vi "lab_21-3.vi"() -> ()   [LabVIEW 2014]
uses:
  <vilib>/addons/Multicore Analysis and Sparse Matrix/Statistics/_statistics/Mean (DBL).vi
  <vilib>/Analysis/NI_AALBase.lvlib
  <vilib>/measure/NI_MABase.lvlib
  <instrlib>/Rohde&Schwarz HMC 804x Power Supplies/Rohde&Schwarz HMC 804x Power Supplies.lvlib
  <vilib>/addons/Multicore Analysis and Sparse Matrix/Statistics/NI_MASM_Statistics.lvlib
panel:
  out "TERMOCOP":cluster{dbl[], dbl[]}(graph)
  out "PT100":cluster{dbl[], dbl[]}(graph)
  in  "tempo tot acquisiz":dbl=100.0
  in  "durata ciclo\n acquisizione dt":dbl=0.1
  in  "freq acquiisizione":dbl=1000.0
  out "0- PULSE":cluster{dbl[], dbl[]}(graph)
  in  "freq quadra":dbl=10.0 format="%0.2p"
  in  "amp quadra":dbl=1.0 format="%0.2p"
  out "Waveform Graph 2":waveform(dbl)(graph)={"t0"=timestamp(0 s since 1904-01-01), "dt"=0.001, "Y"=array[1000 elements]}
  in  "amplitude":dbl=10.0 format="%0.2f"
  in  "Durata impulso":dbl=0.5
  in  "Ritardo":dbl=10.0
  in  "durata tot \nsegnale impulso":dbl=20.0
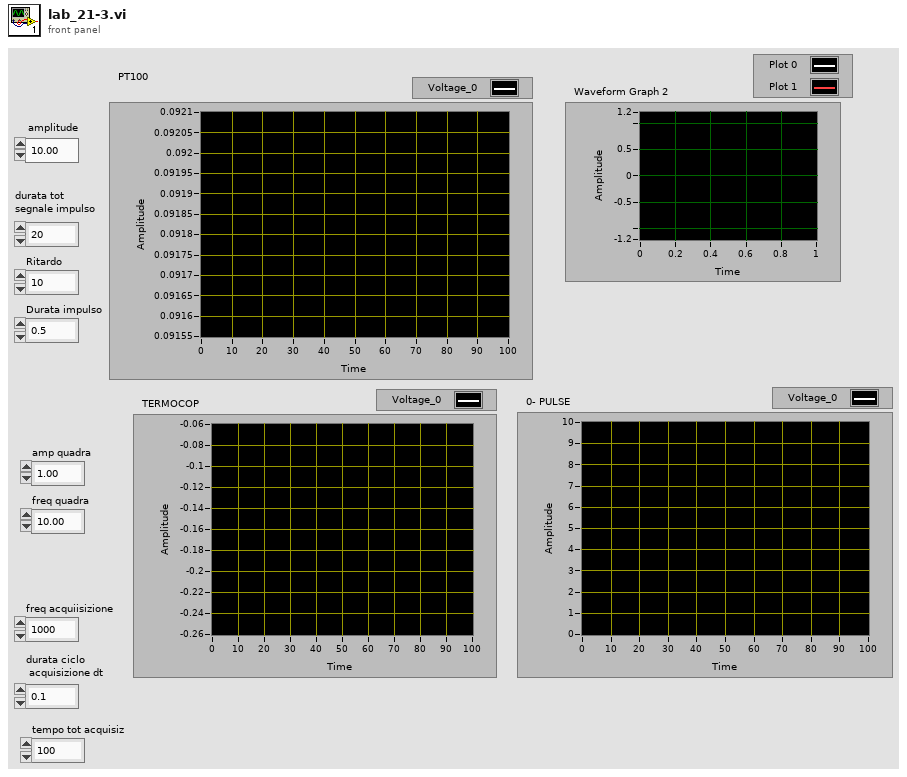
[diagram p1: front panel]
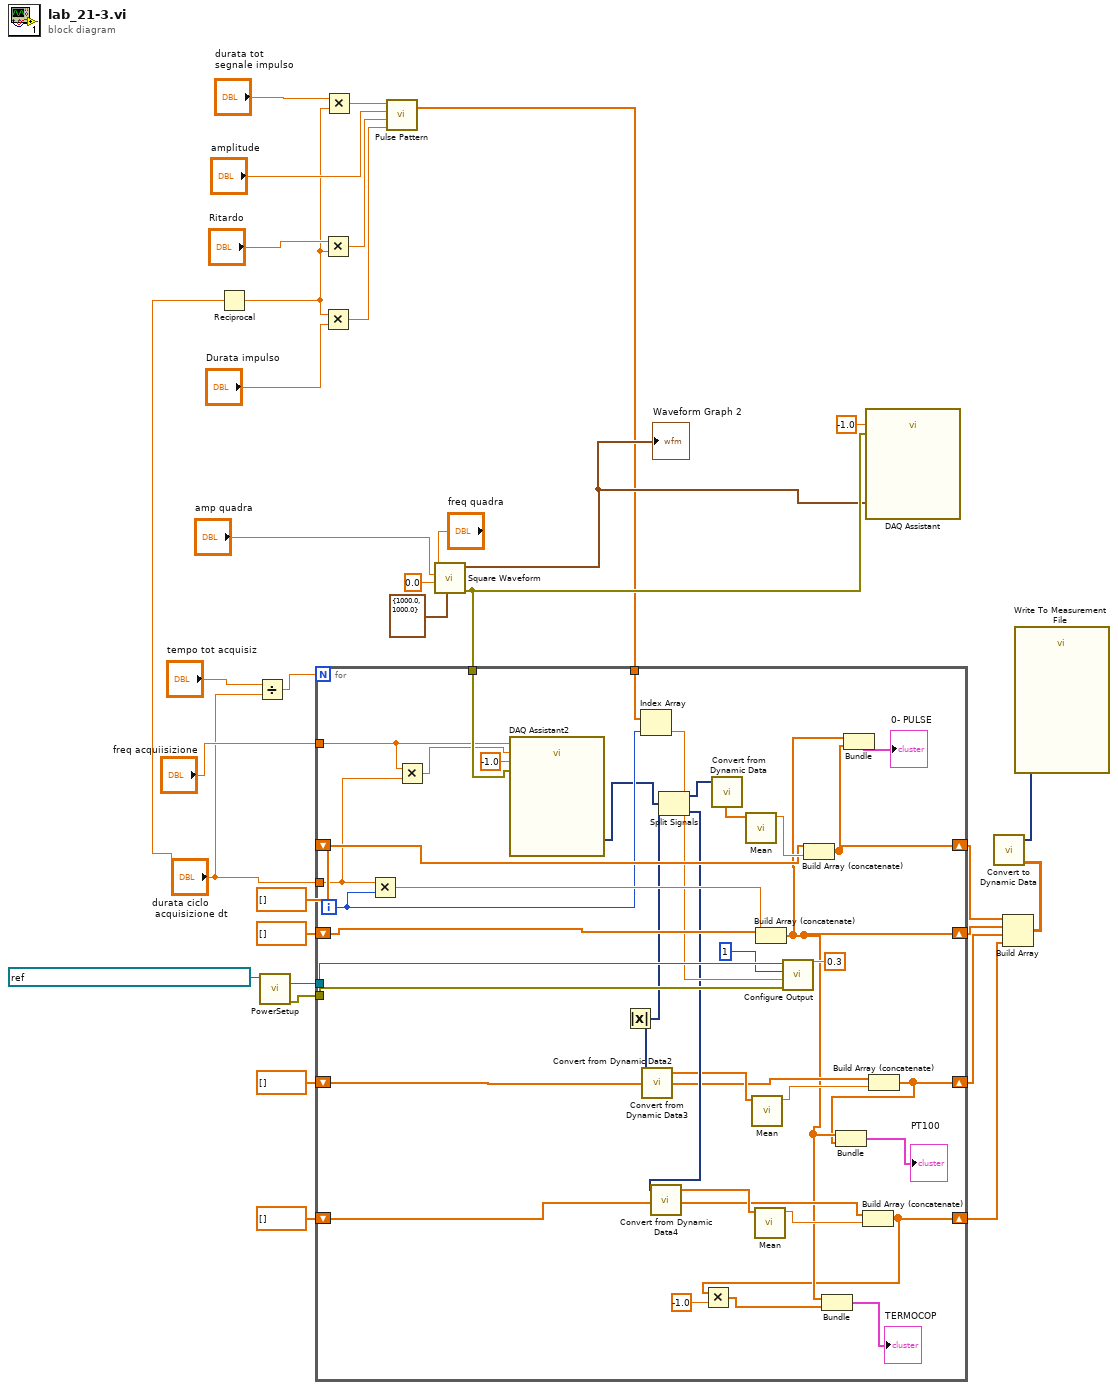
[diagram p0: block diagram]
diagram:
  n1 = Reciprocal(x="durata ciclo\n acquisizione dt") -> (1/x=w11:dbl)
  n2 = Divide(x="tempo tot acquisiz", y="durata ciclo\n acquisizione dt") -> (x/y=w22:dbl)
  n3 = call "PowerSetup.vi"("VISA resource name"=refnum<visa-resource-name> "USB0::0x0AAD::0x0135::035375048::INSTR") -> ("error out"=w9:errorcluster, "VISA resource name out"=w8:refnum<visa-resource-name>)  [unwired: 9 in]
  n4 = Multiply(x="Ritardo", y=w11) -> (x*y=w31:dbl)
  n5 = Multiply(x=w11, y="Durata impulso") -> (x*y=w29:dbl)
  n6 = Multiply(x="durata tot \nsegnale impulso", y=w11) -> (x*y=w25:dbl)
  n7 = call <vilib>:"Pulse Pattern.vi"("width"=w29, "delay"=w31, "amplitude"="amplitude", "samples"=w25) -> ("Pulse Pattern"=w7:dbl[])  [unwired: 1 out]
  n8 = call <vilib>:"Square Waveform.vi"("sampling info"=cluster{"Fs":dbl, "#s":dbl} {"Fs"=1000.0, "#s"=1000.0}, "phase"=0.0, "amplitude"="amp quadra", "frequency"="freq quadra") -> ("error out"=w15:errorcluster, "signal out"=w12:waveform(dbl))  [unwired: 6 in]
  "Waveform Graph 2" <- w12
  n9 = for {
    N: w22 -> [_]
    shift-right: [w60] -> w18
    shift-left: dbl[] [] -> [w68]
    tunnel: "durata ciclo\n acquisizione dt" -> [w62]
    shift-right: [w40] -> w5
    shift-left: dbl[] [] -> [w66]
    tunnel: w15 -> [w64]
    tunnel: "freq acquiisizione" -> [w63]
    tunnel: w9 -> [w59]
    tunnel: w8 -> [w58]
    tunnel: w7 -> [w55]
    shift-right: [w37] -> w3
    shift-left: dbl[] [] -> [w42]
    shift-right: [w39] -> w4
    shift-left: dbl[] [] -> [w43]
    i -> [w56]
    n10 = Multiply(x=w62, y=w56) -> (x*y=w67:dbl)
    n11 = Multiply(x=w63, y=w62) -> (x*y=w61:dbl)
    n12 = call "DAQ Assistant2"("rate"=w63, "number of samples"=w61, "timeout (s)"=-1.0, "error in"=w64) -> ("data"=w51:dynamicdata)  [unwired: 13 in, 2 out]
    n13 = Index Array(array=w55, index=w56) -> (element=w53:dbl)
    n14 = call "Convert from Dynamic Data2"() -> ()  [unwired: 4 in, 1 out]
    n15 = Split Signals(w51) -> (w50:dynamicdata, w49:dynamicdata, w48:dynamicdata)  [unwired: 3 in]
    n16 = Absolute Value(x=w49) -> (abs(x)=w34:dynamicdata)
    n17 = call "Convert from Dynamic Data3"("Dynamic Data Type"=w34) -> ("Array"=w47:dbl[])  [unwired: 3 in]
    n18 = call "Convert from Dynamic Data4"("Dynamic Data Type"=w48) -> ("Array"=w46:dbl[])  [unwired: 3 in]
    n19 = call "Convert from Dynamic Data"("Dynamic Data Type"=w50) -> ("Array"=w52:dbl[])  [unwired: 3 in]
    n20 = call-poly <vilib>:"Mean.vi"("X"=w52) -> ("mean"=w69:dbl)  [unwired: 9 in, 1 out]
    n21 = call-poly <vilib>:"Mean.vi"("X"=w47) -> ("mean"=w45:dbl)  [unwired: 9 in, 1 out]
    n22 = call-poly <vilib>:"Mean.vi"("X"=w46) -> ("mean"=w44:dbl)  [unwired: 9 in, 1 out]
    n23 = Build Array (concatenate)(w66, w67) -> (w40:dbl[])
    n24 = call <instrlib>:"Configure Output.vi"("Current (0.0)"=0.3, "error in (no error)"=w59, "Voltage (0.0)"=w53, "Channel (1)"=1, "VISA resource name"=w58) -> ()  [unwired: 5 in, 2 out]
    n25 = Build Array (concatenate)(w68, w69) -> (w60:dbl[])
    n26 = Bundle(w40, w60) -> (→"0- PULSE":cluster{dbl[], dbl[]})  [unwired: 1 in]
    n27 = Build Array (concatenate)(w42, w44) -> (w37:dbl[])
    n28 = Multiply(x=w37, y=-1.0) -> (x*y=w36:dbl[])
    n29 = Bundle(w40, w36) -> (→"TERMOCOP":cluster{dbl[], dbl[]})  [unwired: 1 in]
    n30 = Build Array (concatenate)(w43, w45) -> (w39:dbl[])
    n31 = Bundle(w40, w39) -> (→"PT100":cluster{dbl[], dbl[]})  [unwired: 1 in]
  }
  n32 = call "DAQ Assistant"("data"=w12, "timeout (s)"=-1.0, "error in"=w15) -> ()  [unwired: 14 in, 3 out]
  n33 = Build Array(w18, w5, w4, w3) -> (w17:dbl[][])
  n34 = call "Convert to Dynamic Data"("2D Array"=w17) -> ("Dynamic Data Type"=w16:dynamicdata)  [unwired: 3 in]
  n35 = call "Write To Measurement File"("Signals"=w16) -> ()  [unwired: 16 in, 3 out]
